vi "modbus数据包解析.vi"(0 "modbus数据":i32[](array[numeric])) -> (3 "湿度1":dbl, 4 "温度1":dbl, 6 "温度2":dbl, 8 "温度3":dbl, 10 "湿度-温度1":dbl, 13 "亮度":dbl, 14 "湿度2":dbl, 15 "湿度-温度2":dbl)   [LabVIEW 2016]
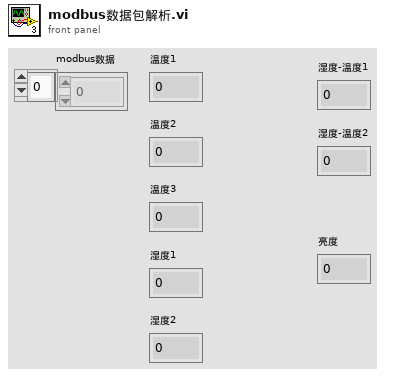
[diagram p1: front panel]
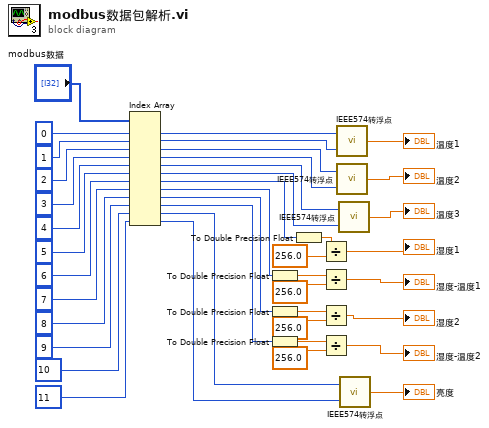
[diagram p0: block diagram]
diagram:
  n1 = Index Array(array="modbus数据", index #1=0 ("索引"), index #2=1 ("索引"), index #3=2 ("索引"), index #4=3 ("索引"), index #5=4 ("索引"), index #6=5 ("索引"), index #7=6 ("索引"), index #8=7 ("索引"), index #9=8 ("索引"), index #10=9 ("索引"), index #11=10 ("索引"), index #12=11 ("索引")) -> (element #1=w8:i32, element #2=w12:i32, element #3=w13:i32, element #4=w14:i32, element #5=w21:i32, element #6=w22:i32, element #7=w27:i32, element #8=w29:i32, element #9=w32:i32, element #10=w33:i32, element #11=w5:i32, element #12=w4:i32)
  n2 = To Double Precision Float(number=w29) -> (double precision float=w26:dbl)
  n3 = To Double Precision Float(number=w32) -> (double precision float=w34:dbl)
  n4 = To Double Precision Float(number=w33) -> (double precision float=w35:dbl)
  n5 = To Double Precision Float(number=w27) -> (double precision float=w28:dbl)
  n6 = Divide(x=w28, y=256.0) -> (x/y=→"湿度1":dbl)
  n7 = Divide(x=w26, y=256.0) -> (x/y=→"湿度-温度1":dbl)
  n8 = Divide(x=w34, y=256.0) -> (x/y=→"湿度2":dbl)
  n9 = Divide(x=w35, y=256.0) -> (x/y=→"湿度-温度2":dbl)
  n10 = call "IEEE574转浮点.vi"("2_byte"=w12, "1_byte"=w8) -> ("Outvalue"=→"温度1":dbl)
  n11 = call "IEEE574转浮点.vi"("2_byte"=w14, "1_byte"=w13) -> ("Outvalue"=→"温度2":dbl)
  n12 = call "IEEE574转浮点.vi"("2_byte"=w22, "1_byte"=w21) -> ("Outvalue"=→"温度3":dbl)
  n13 = call "IEEE574转浮点.vi"("2_byte"=w4, "1_byte"=w5) -> ("Outvalue"=→"亮度":dbl)
